vi "MT Generate PSK System Parameters(map).vi"(0 "samples per symbol (16)":i32=16, 1 "PSK type":u16(ring) items=["normal", "shifted", "offset"], 5 "symbol values":i32[](array[numeric]), 7 "differential PSK":enum16{"disable", "enable"}(ring), 11 "error in (no error)":errorcluster) -> (6 "PSK system parameters":T1 {"PSK type" items=["normal", "shifted", "offset"]; "symbol map" format="%.3f"}, 8 "bits per symbol":i32, 15 "error out":errorcluster)   [LabVIEW 2020, in "niDMT.lvlib"]
doc: "This polymorphic instance calculates parameters for use with either the MT Modulate PSK VI or the MT Demodulate PSK VI. This VI generates the symbol map for PSK-modulated systems. The VI accepts an array of <B>symbol values</B> that explicitly specifies the positions of the symbol map."
uses:
  <vilib>/addons/Modulation/niDMT.lvlib
  <vilib>/addons/Modulation/Digital/Support/Controls/PSK System Parameters.ctl
  <vilib>/addons/Modulation/niAMT.lvlib
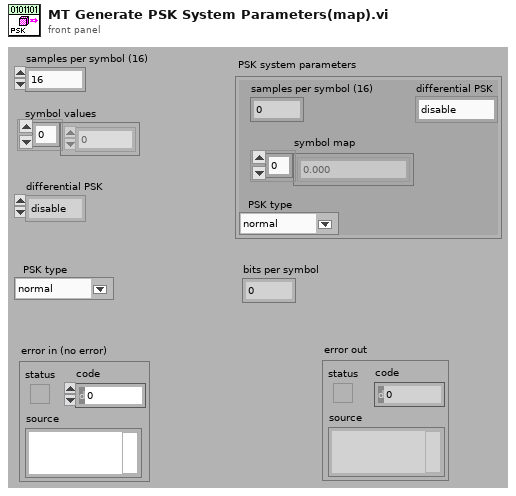
[diagram p1: front panel]
types:
  T1 = cluster{"samples per symbol (16)":i32, "symbol map":cdb[], "differential PSK":enum16{"disable", "enable"}, "PSK type":u16}
  T2 = typedef "niDMT.lvlib/PSK System Parameters.ctl" = cluster{"samples per symbol (16)":i32, "symbol map":cdb[], "differential PSK":enum16{"disable", "enable"}, "PSK type":u16}
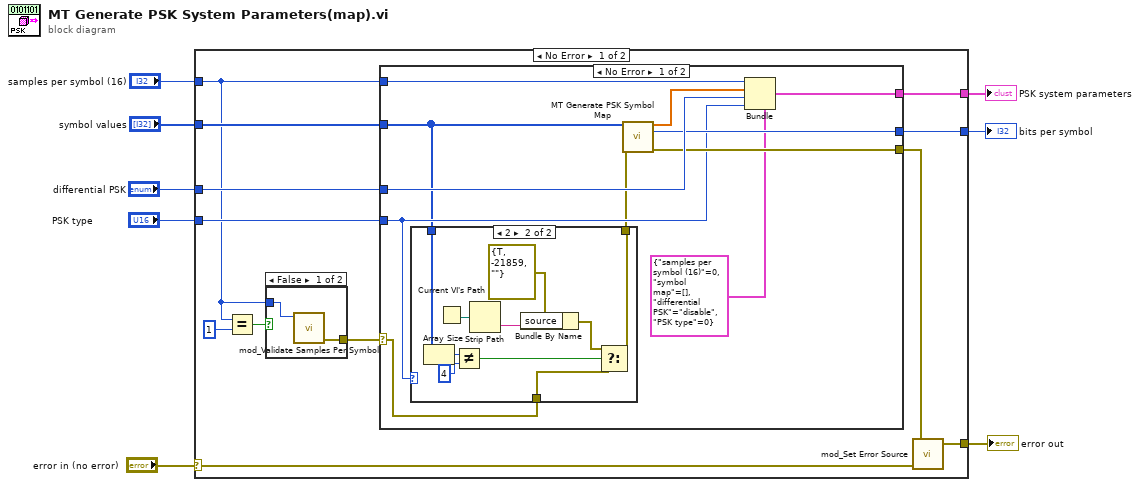
[diagram p0: block diagram]
diagram:
  n1 = case shown="No Error" "error in (no error)" {
    selector: "error in (no error)" -> [w14 w46]
    tunnel: "samples per symbol (16)" -> [w11 _]
    tunnel: "differential PSK" -> [w20 _]
    tunnel: [w19 _] -> w1
    tunnel: "symbol values" -> [w13 _]
    tunnel: "PSK type" -> [w15 _]
    tunnel: [w18 _] -> w4
    tunnel: [w17 w46] -> w3
    frame No Error {
      n2 = Equal?(x=w11, y=1) -> (x = y?=w9:bool)
      n3 = case shown="False" w9 {
        tunnel: w11 -> [w22 _]
        tunnel: [w21 _] -> w12
        frame False {
          n4 = call <vilib>:"mod_Validate Samples Per Symbol.vi"("Samples Per Symbol"=w22) -> ("error out"=w21:errorcluster)  [unwired: 10 out]
        }
        frame True {
        }
      }
      n5 = case shown="No Error" w12 {
        selector: w12 -> [w24 w45]
        tunnel: w20 -> [w33 _]
        tunnel: [w32 _] -> w19
        tunnel: [w30 _] -> w18
        tunnel: [w29 w45] -> w16
        tunnel: w15 -> [w28 _]
        tunnel: w13 -> [w26 _]
        tunnel: w11 -> [w25 _]
        frame No Error {
          n6 = case shown="2" w28 {
            tunnel: [w34 w39] -> w27
            tunnel: w24 -> [w34 w40]
            tunnel: w26 -> [_ w43]
            frame 0, Default {
            }
            frame 2 {
              n7 = Array Size(array=w43) -> (size(s)=w44:i32)
              n8 = Current VI's Path() -> (path=w38:path)
              n9 = Not Equal?(x=w44, y=4) -> (x != y?=w41:bool)
              n10 = Strip Path(path=w38) -> (name=w36:string)  [unwired: 1 out]
              n11 = Bundle By Name(cluster=errorcluster {"status"=TRUE, "code"=-21859, "source"=""} ("error IO"), "source"=w36) -> (w35:errorcluster)
              n12 = Select(t=w35, s=w41, f=w40) -> (s? t:f=w39:errorcluster)
            }
          }
          n13 = call <vilib>:"MT Generate PSK Symbol Map.vi"("symbol values"=w26, "error in (no error)"=w27) -> ("symbol map"=w31:cdb[], "bits per symbol"=w30:i32, "error out"=w29:errorcluster)  [unwired: 11 out]
          n14 = Bundle(cluster=T2 {"samples per symbol (16)"=0, "symbol map"=[], "differential PSK"=enum."disable", "PSK type"=0} ("PSK system parameters"), "samples per symbol (16)"=w25, "symbol map"=w31, "differential PSK"=w33, "PSK type"=w28) -> (w32:T2)
        }
        frame Error {
        }
      }
      n15 = call <vilib>:"mod_Set Error Source.vi"("initial error in (no error)"=w14, "final error in (no error)"=w16) -> ("error out"=w17:errorcluster)  [unwired: 3 out]
    }
    frame Error {
    }
  }
  "PSK system parameters" <- w1
  "bits per symbol" <- w4
  "error out" <- w3
